vi "Read Repetitions.vi"(8 "error in (no error)":errorcluster, 11 "Schedule Cell in":refnum<class "Schedule Cell.lvclass">) -> (0 "error out":errorcluster, 2 "Repetitions":u32=1 min=1, 3 "Schedule Cell out":refnum<class "Schedule Cell.lvclass">)   [LabVIEW 2020, in "Run Utilities.lvlib" / "Schedule Cell.lvclass"]
uses:
  Schedule Cell.lvclass
  Schedule Cell.lvclass/Schedule Cell.ctl
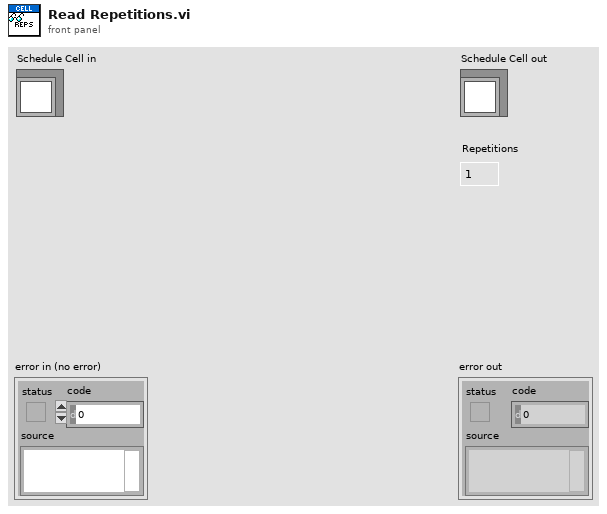
[diagram p1: front panel]
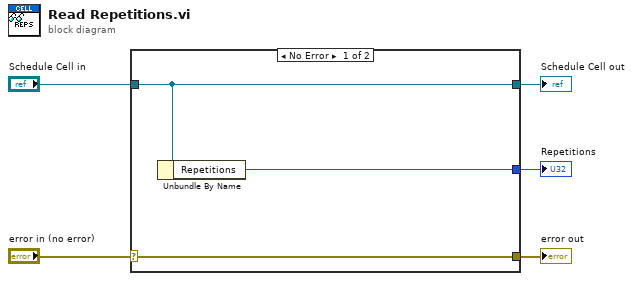
[diagram p0: block diagram]
diagram:
  n1 = case shown="No Error" "error in (no error)" {
    selector: "error in (no error)" -> [w8 w9]
    tunnel: [w8 w9] -> w4
    tunnel: [w7 w10] -> w2
    tunnel: "Schedule Cell in" -> [w7 w10]
    tunnel: [w6 _] -> w1
    frame No Error {
      n2 = Unbundle By Name(w7) -> ("Repetitions"=w6:u32)
    }
    frame Error {
    }
  }
  "error out" <- w4
  "Schedule Cell out" <- w2
  "Repetitions" <- w1
